vi "Mini-Circuits-RF-Switch.vi"(6 "RFSW State":T1=enum."1", 7 "RFSW Letter":T2, 11 "Switch 1 SN":string(combo)) -> (0 "Error Out":errorcluster, 3 "SWA":bool, 4 "Model_Name SW1":string)   [LabVIEW 2020]
uses:
  Subs/RFSW Letter.ctl
  Subs/RFSW State.ctl
  Subs/Mini-Circuits-RF-Switch.ctl
  <vilib>/Utility/file.llb/Read Delimited Spreadsheet (string).vi
  <vilib>/Utility/file.llb/Write Delimited Spreadsheet (string).vi
panel:
  out "ExeName":string
  out "Test Config Path Out":path
  in  "Set_Switch":bool
  out "current test path":string[](array[string])
  out "test-paths":string[](array[string])=["CMN4-RX1", "CMN4-RX2", "CMN4-NF1", "CMN4-NF2", "UVL-TX1", "UVL-TX2", "WBHD-RX1", "WBHD-RX2", "WBHD-RX3", "WBHD-NF1", "WBHD-NF2", "WBHD-NF3", "WBHD-TX1", "WBHD-TX2", "WBHD-TX3", "NB-RX1", "NB-RX2", "NB-NF1", "NB-NF2"]
  out "State":string="Exit"
  out "INI Path":path=path "C:/Users/J54147.NORTHGRUM/OneDrive - NGC/Documents/LabVIEW Data/Config Files/mcl_RF_Switch_Main_GUI_Config.ini"
  in  "Tab Control":enum32{"Main", "Configuration"}(tab)
  in  "Stop Button":bool
  in  "Load Config":bool
  in  "Save Config":bool
  in  "Get_State":bool
  in  "Set Path":bool
  in  "Test Path":T3
  in  "Switch 2 SN":string(combo)
  out "Model_Name SW2":string
  out "SW B":bool
  in  "SW 2A":u8(knob)=1 min=1 max=7 step=1 scale=1.0..6.0
  in  "SW 1B":u8(knob)=1 min=1 max=7 step=1 scale=1.0..6.0
  in  "SW 1A":u8(knob)=1 min=1 max=7 step=1 scale=1.0..6.0
  in  "Paths Config":string[][](table)
  in  "Test Config Path":path
  # "AMCTR RF SWITCH UTILITY"
  # "v.1.0"
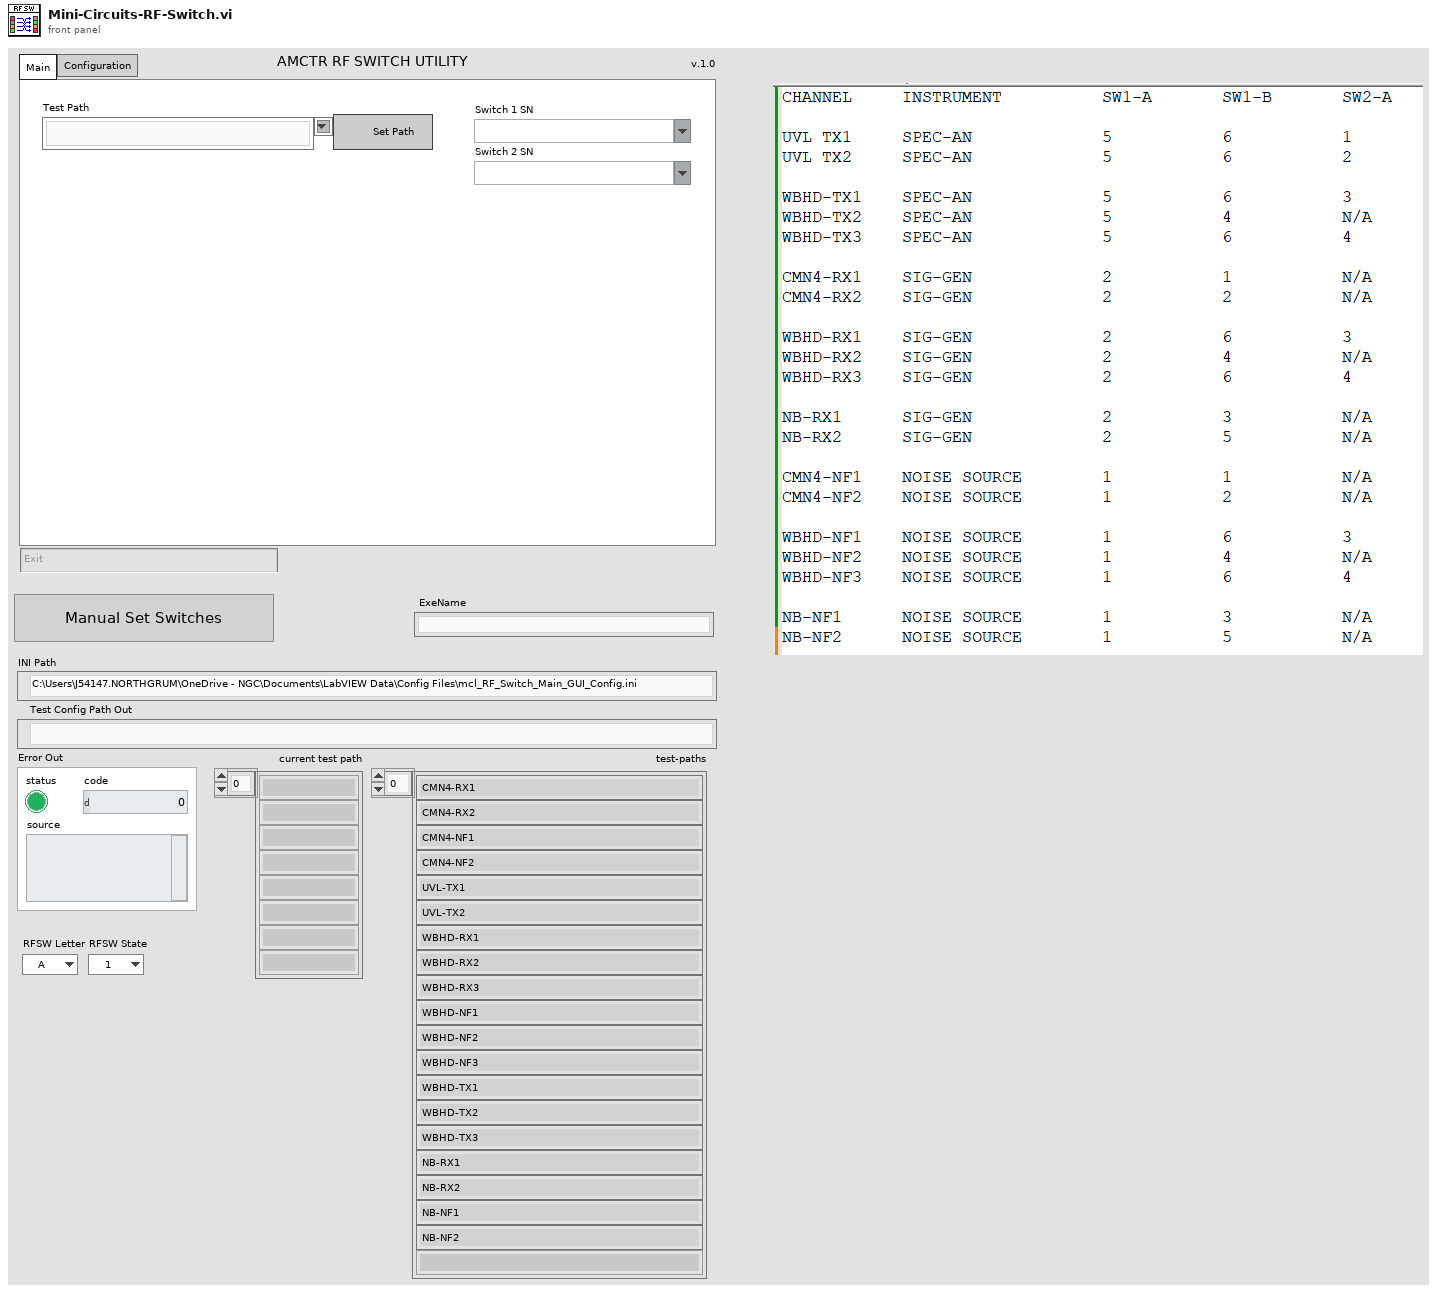
[diagram p1: front panel]
types:
  T1 = typedef "RFSW State.ctl" = enum16{"0", "1", "2", "3", "4", "5", "6"}
  T2 = typedef "RFSW Letter.ctl" = enum16{"A", "B"}
  T3 = typedef "Mini-Circuits-RF-Switch.ctl" = string
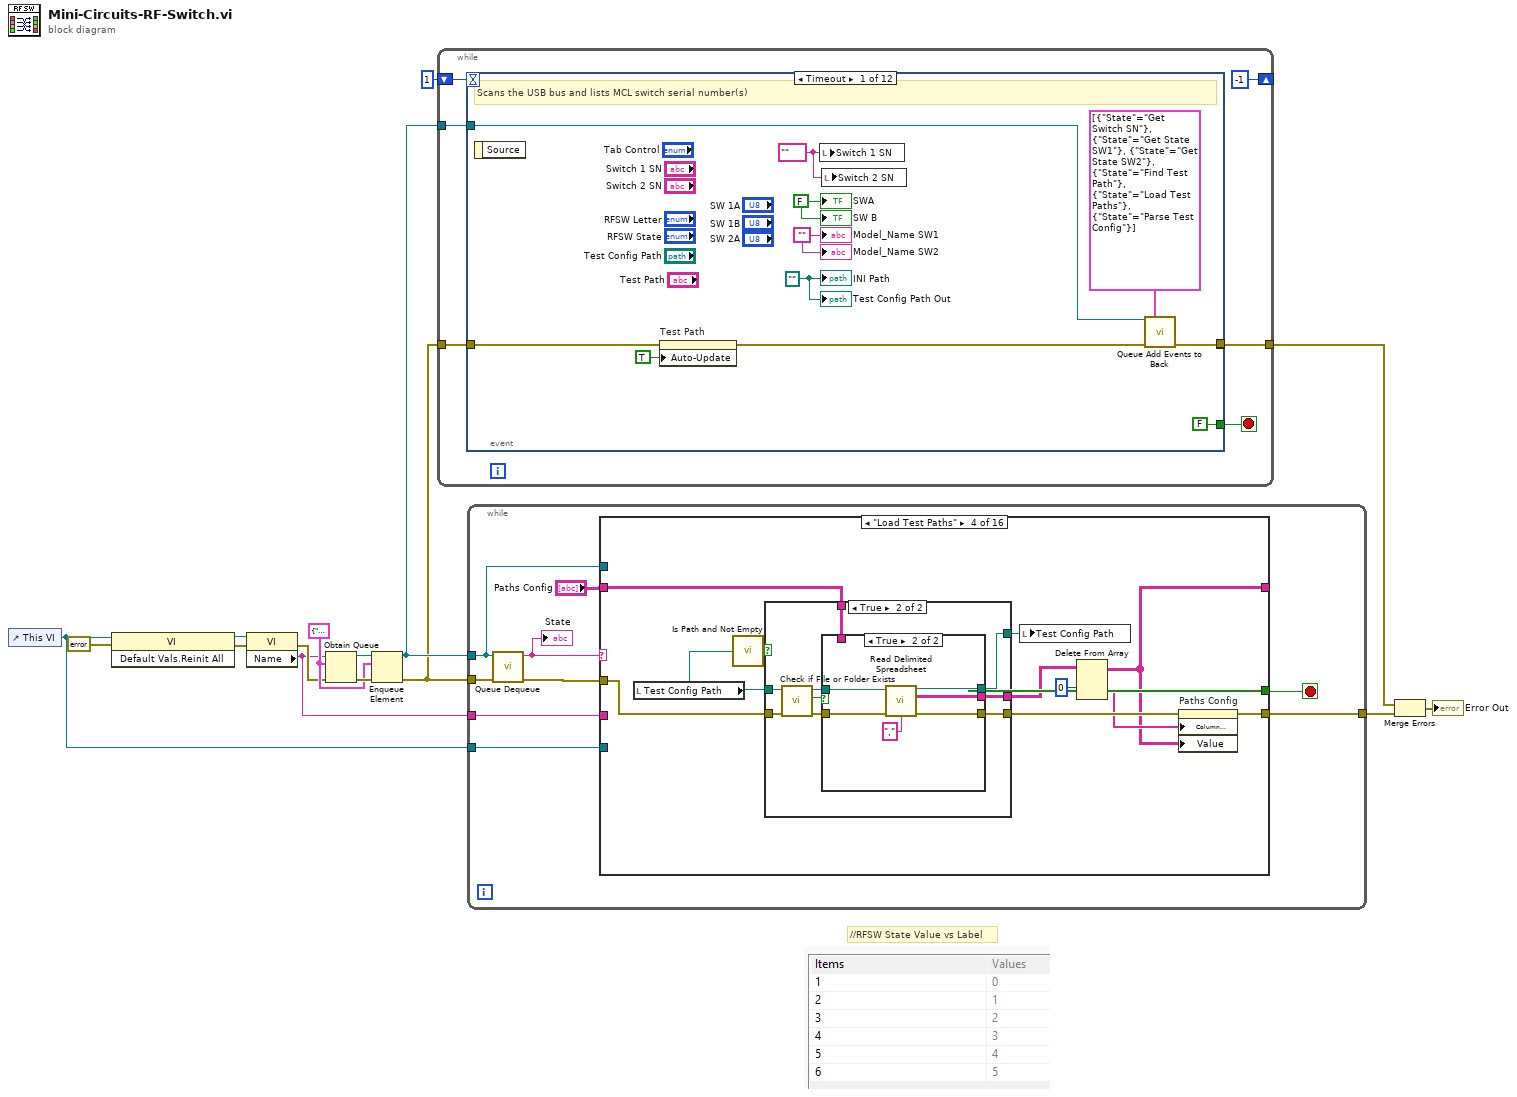
[diagram p0: block diagram]
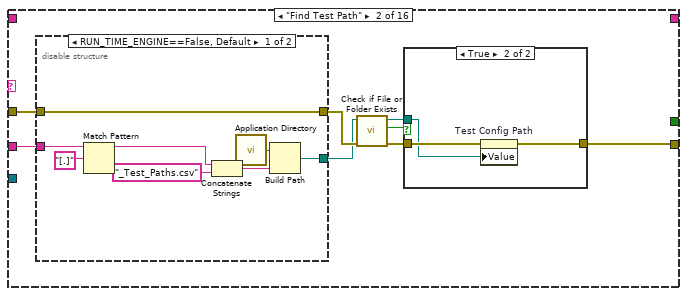
[diagram p3: hidden frame]
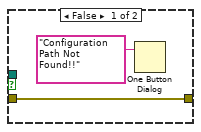
[diagram p4: hidden frame]
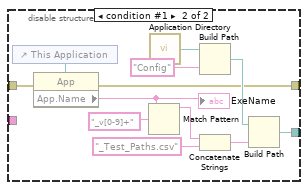
[diagram p5: hidden frame]
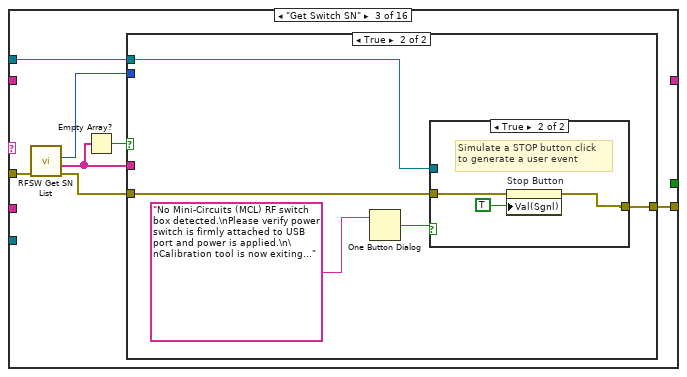
[diagram p6: hidden frame]
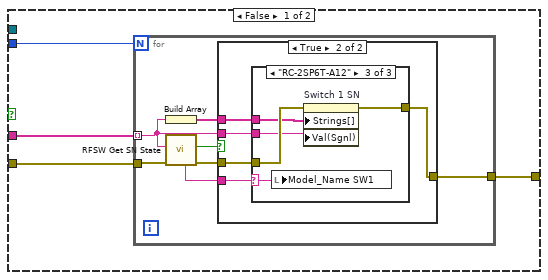
[diagram p7: hidden frame]
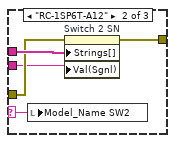
[diagram p10: hidden frame]
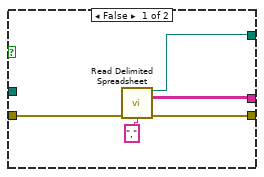
[diagram p12: hidden frame]
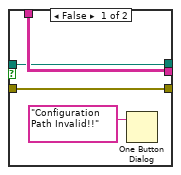
[diagram p13: hidden frame]
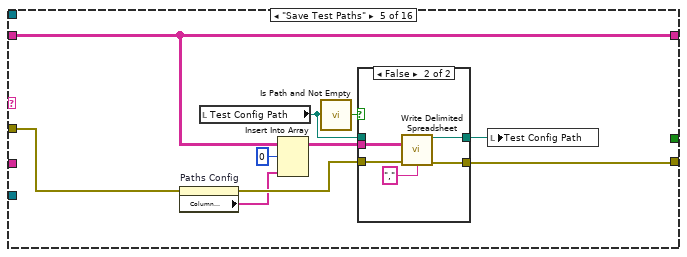
[diagram p14: hidden frame]
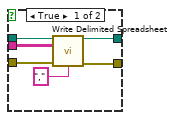
[diagram p15: hidden frame]
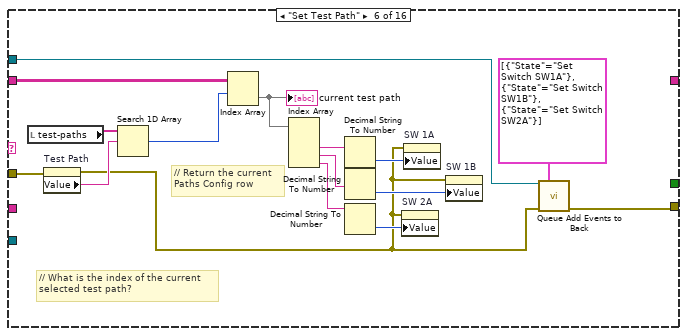
[diagram p16: hidden frame]
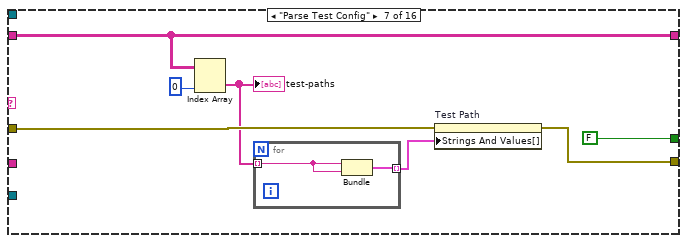
[diagram p17: hidden frame]
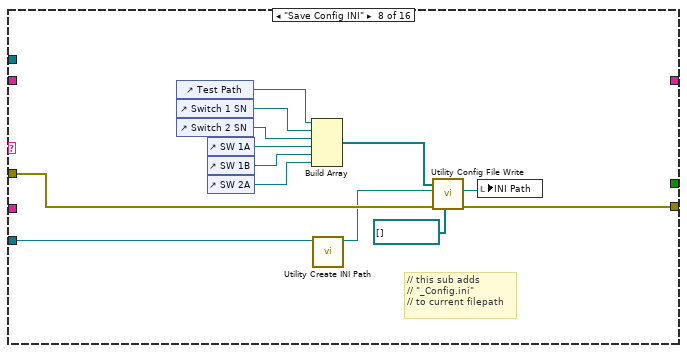
[diagram p18: hidden frame]
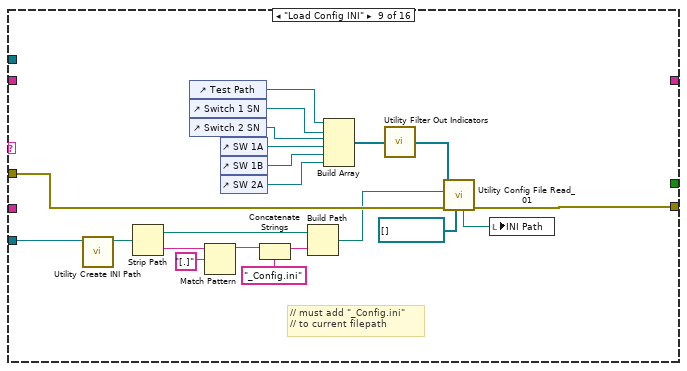
[diagram p19: hidden frame]
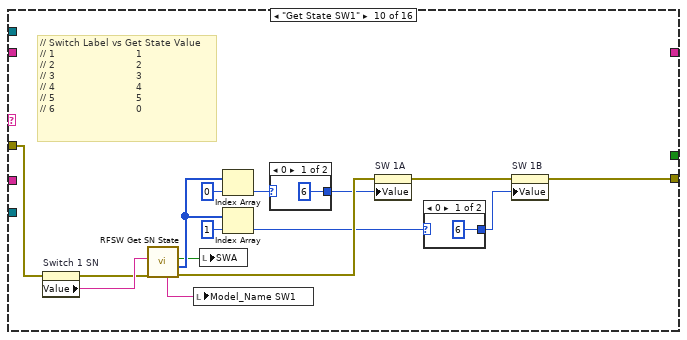
[diagram p20: hidden frame]
diagram:
  w11 = cluster{"State":string, "Data":variant} {"State"="", "Data"=variant} ("Cluster")
  # "//RFSW State Value vs Label"
  n1 = control-ref of="This VI"() -> (w4:refnum<vi>)
  n2 = invoke class="VI" method="Default Vals.Reinit All"(reference=w4, error in=errorcluster {"status"=FALSE, "code"=0, "source"=""} ("Error In")) -> (reference out=w8:refnum<vi>, error out=w7:errorcluster)  [unwired: 1 in, 1 out]
  n3 = property class="VI"(reference=w8, error in=w7) -> (error out=w10:errorcluster, "Name"=w1:string)  [unwired: 1 out]
  n4 = Obtain Queue(name (unnamed)=w1, element data type=w11, error in (no error)=w10) -> (queue out=w12:refnum<queue>, error out=w13:errorcluster)  [unwired: 2 in, 1 out]
  n5 = Enqueue Element(queue=w12, element=w11, error in (no error)=w13) -> (queue out=w9:refnum<queue>, error out=w2:errorcluster)  [unwired: 1 in, 1 out]
  n6 = while {
    tunnel: w2 -> [w21]
    tunnel: [w20] -> w15
    shift-right: [-1] -> _
    shift-left: 1 -> [w18]
    tunnel: w9 -> [w16]
    stop <- w19 stop-if-true
    n7 = event shown="[0] Timeout" {
      selector: _ -> [_ _ _ _ _ _ _ _ _ _ _ _]
      dyn-events: _ -> [_ _ _ _ _ _ _ _ _ _ _ _]
      timeout: w18 -> [_ _ _ _ _ _ _ _ _ _ _ _]
      tunnel: w21 -> [w24 w35 w44 w52 w58 w69 w73 w77 w81 w85 w91 w103]
      tunnel: [_ w34 w43 w51 w57 w68 w71 w75 w79 w84 w90 w102] -> w20
      tunnel: [FALSE _ _ FALSE FALSE FALSE _ _ _ TRUE TRUE TRUE] -> w19
      tunnel: w16 -> [w29 w36 w45 w53 w59 w66 w72 w76 w80 w86 w92 w104]
      tunnel: [w28 _ _ _ _ _ _ _ _ _ _ _] -> _
      event Timeout {
        w25 = "" ("Switch 1 SN")
        w26 = path ""
        w30 = ""
        w31 = FALSE ("Connected?")
        # "Scans the USB bus and lists MCL switch serial number(s)"
        n8 = event-data() -> ()  [unwired: 1 in, 1 out]
        n9 = property on="Test Path" class="CmbBox (strict)"(error in=w24, "Auto-Update"=TRUE ("Auto-Update From Typedef")) -> (error out=w23:errorcluster)  [unwired: 1 in, 1 out]
        n10 = local write "Switch 1 SN"(w25) -> ()
        n11 = local write "Switch 2 SN"(w25) -> ()
        n12 = call "Queue Add Events to Back.vi"("Queue In"=w29, "State Array"=cluster{"State":string}[] [{"State"="Get Switch SN"}, {"State"="Get State SW1"}, {"State"="Get State SW2"}, {"State"="Find Test Path"}, {"State"="Load Test Paths"}, {"State"="Parse Test Config"}], "Error In"=w23) -> ("Error Out"=w28:errorcluster)  [unwired: 11 in, 1 out]
        "Model_Name SW1" <- w30
        "SWA" <- w31
        "INI Path" <- w26
        "SW B" <- w31
        "Model_Name SW2" <- w30
        "Test Config Path Out" <- w26
      }
      event "Save Config": Value Change {
        n13 = event-data() -> ("NewVal"=w33:bool)  [unwired: 1 in]
        n14 = case shown="True" w33 {
          tunnel: w36 -> [_ w40]
          tunnel: w35 -> [w37 w39]
          tunnel: [w37 w38] -> w34
          frame False {
          }
          frame True {
            n15 = call "Queue Add Events to Back.vi"("Queue In"=w40, "State Array"=cluster{"State":string}[] [{"State"="Save Config INI"}, {"State"="Save Test Paths"}], "Error In"=w39) -> ("Error Out"=w38:errorcluster)  [unwired: 11 in, 1 out]
          }
        }
      }
      event "Load Config": Value Change {
        n16 = event-data() -> ("NewVal"=w42:bool)  [unwired: 1 in]
        n17 = case shown="True" w42 {
          tunnel: w45 -> [_ w49]
          tunnel: w44 -> [w46 w48]
          tunnel: [w46 w47] -> w43
          frame False {
          }
          frame True {
            n18 = call "Queue Add Events to Back.vi"("Queue In"=w49, "State Array"=cluster{"State":string}[] [{"State"="Load Config INI"}], "Error In"=w48) -> ("Error Out"=w47:errorcluster)  [unwired: 11 in, 1 out]
          }
        }
      }
      event "Set_Switch": Value Change {
        n19 = event-data() -> ()  [unwired: 1 in, 1 out]
        n20 = call "Queue Add Events to Back.vi"("Queue In"=w53, "State Array"=cluster{"State":string}[] [{"State"="Set Switch SW1A"}, {"State"="Set Switch SW1B"}, {"State"="Set Switch SW2A"}], "Error In"=w52) -> ("Error Out"=w51:errorcluster)  [unwired: 11 in, 1 out]
      }
      event "Set Path": Value Change {
        n21 = event-data() -> ("NewVal"=w56:bool)  [unwired: 1 in]
        n22 = case shown="True" w56 {
          tunnel: w59 -> [_ w64]
          tunnel: w58 -> [w61 w63]
          tunnel: [w61 w62] -> w57
          frame False {
          }
          frame True {
            n23 = call "Queue Add Events to Back.vi"("Queue In"=w64, "State Array"=cluster{"State":string}[] [{"State"="Set Test Path"}], "Error In"=w63) -> ("Error Out"=w62:errorcluster)  [unwired: 11 in, 1 out]
          }
        }
      }
      event "Get_State": Value Change {
        n24 = event-data() -> ()  [unwired: 1 in, 1 out]
        n25 = call "Queue Add Events to Back.vi"("Queue In"=w66, "State Array"=cluster{"State":string}[] [{"State"="Get State SW1"}, {"State"="Get State SW2"}], "Error In"=w69) -> ("Error Out"=w68:errorcluster)  [unwired: 11 in, 1 out]
      }
      event "SW 1A": Value Change {
        n26 = event-data() -> ()  [unwired: 1 in, 1 out]
        n27 = call "Queue Add Events to Back.vi"("Queue In"=w72, "State Array"=cluster{"State":string}[] [{"State"="Set Switch SW1A"}], "Error In"=w73) -> ("Error Out"=w71:errorcluster)  [unwired: 11 in, 1 out]
      }
      event "SW 1B": Value Change {
        n28 = event-data() -> ()  [unwired: 1 in, 1 out]
        n29 = call "Queue Add Events to Back.vi"("Queue In"=w76, "State Array"=cluster{"State":string}[] [{"State"="Set Switch SW1B"}], "Error In"=w77) -> ("Error Out"=w75:errorcluster)  [unwired: 11 in, 1 out]
      }
      event "SW 2A": Value Change {
        n30 = event-data() -> ()  [unwired: 1 in, 1 out]
        n31 = call "Queue Add Events to Back.vi"("Queue In"=w80, "State Array"=cluster{"State":string}[] [{"State"="Set Switch SW2A"}], "Error In"=w81) -> ("Error Out"=w79:errorcluster)  [unwired: 11 in, 1 out]
      }
      event Panel Close? {
        n32 = event-data() -> ()  [unwired: 1 in, 1 out]
        n33 = call "Queue Add Events to Back.vi"("Queue In"=w86, "State Array"=cluster{"State":string}[] [{"State"="Save Config INI"}, {"State"="Save Test Paths"}, {"State"="Exit"}], "Error In"=w85) -> ("Error Out"=w84:errorcluster)  [unwired: 11 in, 1 out]
        n34 = event-data("Discard?"=TRUE) -> ()  [unwired: 1 in, 1 out]
      }
      event "Stop Button": Value Change {
        n35 = event-data() -> ("NewVal"=w89:bool)  [unwired: 1 in]
        n36 = case shown="True" w89 {
          tunnel: w92 -> [_ w100]
          tunnel: w91 -> [w94 w99]
          tunnel: [w94 w96] -> w90
          frame False {
          }
          frame True {
            n37 = call "Queue Add Events to Back.vi"("Queue In"=w100, "State Array"=cluster{"State":string}[] [{"State"="Save Config INI"}, {"State"="Save Test Paths"}, {"State"="Exit"}], "Error In"=w99) -> ("Error Out"=w97:errorcluster)  [unwired: 11 in, 1 out]
            n38 = property on="Stop Button" class="Bool (strict)"(error in=w97, "Value"=FALSE ("Stop Button")) -> (error out=w96:errorcluster)  [unwired: 1 in, 1 out]
          }
        }
      }
      event Application Instance Close {
        n39 = event-data() -> ()  [unwired: 1 in, 1 out]
        n40 = call "Queue Add Events to Back.vi"("Queue In"=w104, "State Array"=cluster{"State":string}[] [{"State"="Save Config INI"}, {"State"="Save Test Paths"}, {"State"="Exit"}], "Error In"=w103) -> ("Error Out"=w102:errorcluster)  [unwired: 11 in, 1 out]
      }
    }
  }
  n41 = while {
    tunnel: w2 -> [w114]
    tunnel: w9 -> [w110]
    tunnel: w4 -> [w109]
    tunnel: [w107] -> w5
    tunnel: w1 -> [w106]
    stop <- w112 stop-if-true
    n42 = call "Queue Dequeue.vi"("Error In"=w114, "Queue In"=w110) -> ("Error Out"=w111:errorcluster, "State"=w113:string)  [unwired: 7 in, 1 out]
    "State" <- w113
    n43 = case shown="\"Load Test Paths\"" w113 {
      tunnel: "Paths Config" -> [_ _ _ w197 w237 w261 w266 _ _ _ _ _ _ _ _ _]
      tunnel: [_ _ _ _ _ _ FALSE _ _ _ _ _ _ _ _ w384] -> w112
      tunnel: w111 -> [w115 w123 w155 w198 w235 w264 w269 w286 w307 w313 w330 w344 w352 w365 w373 w382]
      tunnel: w110 -> [_ _ w149 _ _ w250 _ _ _ _ _ _ _ _ _ w385]
      tunnel: w109 -> [_ _ _ _ _ _ _ w285 w306 _ _ _ _ _ _ _]
      tunnel: [_ _ _ w193 w237 _ w266 _ _ _ _ _ _ _ _ _] -> _
      tunnel: [w115 w122 w152 w200 w236 w249 w265 w284 w305 w308 w327 w341 w351 w362 w372 w383] -> w107
      tunnel: w106 -> [_ w121 _ _ _ _ _ _ _ _ _ _ _ _ _ _]
      frame "Timeout", Default {
      }
      frame "Find Test Path" {
        n44 = disable-structure shown="RUN_TIME_ENGINE==False, Default" {
          disable-tunnel: w121 -> [w131 _]
          disable-tunnel: [w134 w146] -> w118
          disable-tunnel: w123 -> [w129 w139]
          disable-tunnel: [w129 w137] -> w120
          frame condition #0 (active) {
            n45 = Match Pattern(string=w131, regular expression="[.]" ("search string")) -> (before substring=w130:string)  [unwired: 1 in, 3 out]
            n46 = Concatenate Strings(w130, "_Test_Paths.csv" ("string")) -> (w136:string)
            n47 = call <vilib>:"Application Directory.vi"() -> ("Application Directory"=w133:path)
            n48 = Build Path(base path=w133, name or relative path=w136) -> (appended path=w134:path)
          }
          frame condition #1 {
            n49 = control-ref of="This Application"() -> (w138:refnum<vi>)
            n50 = property class="App"(reference=w138, error in=w139) -> (error out=w137:errorcluster, "App.Name"=w140:string)  [unwired: 1 out]
            "ExeName" <- w140
            n51 = Match Pattern(string=w140, regular expression="_v[0-9]+" ("search string")) -> (before substring=w141:string)  [unwired: 1 in, 3 out]
            n52 = call <vilib>:"Application Directory.vi"() -> ("Application Directory"=w145:path)
            n53 = Build Path(base path=w145, name or relative path="Config") -> (appended path=w143:path)
            n54 = Concatenate Strings(w141, "_Test_Paths.csv" ("string")) -> (w148:string)
            n55 = Build Path(base path=w143, name or relative path=w148) -> (appended path=w146:path)
          }
        }
        n56 = call <vilib>:"Check if File or Folder Exists.vi"("error in (no error)"=w120, "path"=w118) -> ("error out"=w119:errorcluster, "file or folder exists?"=w117:bool, "dup path"=w116:path)  [unwired: 7 in]
        n57 = case shown="True" w117 {
          tunnel: [w125 w128] -> w122
          tunnel: w119 -> [w125 w127]
          tunnel: w116 -> [_ w126]
          frame False {
            n58 = One Button Dialog(message="Configuration Path Not Found!!") -> ()  [unwired: 1 in, 1 out]
          }
          frame True {
            n59 = property on="Test Config Path" class="Path"(error in=w127, "Value"=w126) -> (error out=w128:errorcluster)  [unwired: 1 in, 1 out]
          }
        }
      }
      frame "Get Switch SN" {
        n60 = call "RFSW Get SN List.vi"("Error_In"=w155) -> ("Error_Out"=w154:errorcluster, "SN_Array"=w151:string[], "Num_Switches"=w153:i32)  [unwired: 7 in, 1 out]
        n61 = Empty Array?(array=w151) -> (empty?=w150:bool)
        n62 = case shown="True" w150 {
          tunnel: w154 -> [w159 w186]
          tunnel: w153 -> [w158 _]
          tunnel: [w157 w188] -> w152
          tunnel: w151 -> [w156 _]
          tunnel: w149 -> [_ w187]
          frame False {
            n63 = for {
              N: w158 -> [_]
              tunnel: w156 -> [w160] mode=indexing
              tunnel: w159 -> [w165]
              tunnel: [w163] -> w157
              n64 = Build Array(w160) -> (w166:string[])
              n65 = call "RFSW Get SN State.vi"("error in (no error)"=w165, "SN"=w160) -> ("error out"=w164:errorcluster, "Connected?"=w161:bool, "Model Name"=w162:string)  [unwired: 5 in, 2 out]
              n66 = case shown="True" w161 {
                tunnel: w166 -> [_ w172]
                tunnel: w164 -> [w167 w171]
                tunnel: [w167 w170] -> w163
                tunnel: w162 -> [_ w169]
                tunnel: w160 -> [_ w168]
                frame False {
                }
                frame True {
                  n67 = case shown="\"RC-2SP6T-A12\"" w169 {
                    selector: w169 -> [_ w178 w183]
                    tunnel: w172 -> [_ w177 w181]
                    tunnel: w171 -> [w173 w176 w182]
                    tunnel: [w173 w175 w180] -> w170
                    tunnel: w168 -> [_ w174 w179]
                    frame Default {
                    }
                    frame "RC-1SP6T-A12" {
                      n68 = local write "Model_Name SW2"(w178) -> ()
                      n69 = property on="Switch 2 SN" class="CmbBox"(error in=w176, "Strings[]"=w177, "Val(Sgnl)"=w174) -> (error out=w175:errorcluster)  [unwired: 1 in, 1 out]
                    }
                    frame "RC-2SP6T-A12" {
                      n70 = local write "Model_Name SW1"(w183) -> ()
                      n71 = property on="Switch 1 SN" class="CmbBox"(error in=w182, "Strings[]"=w181, "Val(Sgnl)"=w179) -> (error out=w180:errorcluster)  [unwired: 1 in, 1 out]
                    }
                  }
                }
              }
            }
          }
          frame True {
            n72 = One Button Dialog(message="No Mini-Circuits (MCL) RF switch box detected.\nPlease verify power switch is firmly attached to USB port and power is applied.\n\nCalibration tool is now exiting...") -> (true=w185:bool)  [unwired: 1 in]
            n73 = case shown="True" w185 {
              tunnel: [w189 w191] -> w188
              tunnel: w187 -> [_ _]
              tunnel: w186 -> [w189 w192]
              frame False {
              }
              frame True {
                # "Simulate a STOP button click\nto generate a user event"
                n74 = property on="Stop Button" class="Bool (strict)"(error in=w192, "Val(Sgnl)"=TRUE ("Value (Signaling)")) -> (error out=w191:errorcluster)  [unwired: 1 in, 1 out]
              }
            }
          }
        }
      }
      frame "Load Test Paths" {
        n75 = local read "Test Config Path"() -> (w195:path)
        n76 = call <vilib>:"Is Path and Not Empty.vi"("path"=w195) -> ("Is Path and Not Empty?"=w196:bool)  [unwired: 4 in]
        n77 = case shown="True" w196 {
          tunnel: [w205 w217] -> w203
          tunnel: [w206 w216] -> w201
          tunnel: w198 -> [w207 w215]
          tunnel: w197 -> [_ w212]
          tunnel: w195 -> [_ w211]
          tunnel: [w204 w209] -> w194
          frame False {
            n78 = call-poly <vilib>:"Read Delimited Spreadsheet.vi"("error in (no error)"=w207, "delimiter (\\t)"="," ("delimiter (\\t)")) -> ("new file path (Not A Path if cancelled)"=w204:path, "all rows"=w205:string[][], "error out"=w206:errorcluster)  [unwired: 8 in, 3 out]
          }
          frame True {
            n79 = call <vilib>:"Check if File or Folder Exists.vi"("error in (no error)"=w215, "path"=w211) -> ("error out"=w214:errorcluster, "file or folder exists?"=w213:bool, "dup path"=w210:path)  [unwired: 7 in]
            n80 = case shown="True" w213 {
              tunnel: [w220 w226] -> w217
              tunnel: [w221 w225] -> w216
              tunnel: w214 -> [w221 w224]
              tunnel: w212 -> [w220 _]
              tunnel: w210 -> [w218 w223]
              tunnel: [w218 w222] -> w209
              frame False {
                n81 = One Button Dialog(message="Configuration Path Invalid!!") -> ()  [unwired: 1 in, 1 out]
              }
              frame True {
                n82 = call-poly <vilib>:"Read Delimited Spreadsheet.vi"("file path (dialog if empty)"=w223, "error in (no error)"=w224, "delimiter (\\t)"="," ("delimiter (\\t)")) -> ("new file path (Not A Path if cancelled)"=w222:path, "all rows"=w226:string[][], "error out"=w225:errorcluster)  [unwired: 7 in, 3 out]
              }
            }
          }
        }
        n83 = local write "Test Config Path"(w194) -> ()
        n84 = Delete From Array(array=w203, index (row)=0) -> (deleted portion=w199:string[], array with subset deleted=w193:string[][])  [unwired: 2 in]
        n85 = property on="Paths Config" class="Tbl (strict)"(error in=w201, "Column Headers[]"=w199, "Value"=w193) -> (error out=w200:errorcluster)  [unwired: 1 in, 1 out]
      }
      frame "Save Test Paths" {
        n86 = property on="Paths Config" class="Tbl (strict)"(error in=w235) -> (error out=w233:errorcluster, "Column Headers[]"=w232:string[])  [unwired: 1 in, 1 out]
        n87 = local read "Test Config Path"() -> (w234:path)
        n88 = Insert Into Array(array=w237, index (row)=0, new element=w232) -> (w230:string[][])  [unwired: 1 in]
        n89 = call <vilib>:"Is Path and Not Empty.vi"("path"=w234) -> ("Is Path and Not Empty?"=w229:bool)  [unwired: 4 in]
        n90 = case shown="False" w229 {
          tunnel: [w243 w248] -> w236
          tunnel: w234 -> [w242 _]
          tunnel: w233 -> [w240 w246]
          tunnel: w230 -> [w239 w245]
          tunnel: [w238 w244] -> w228
          frame True {
            n91 = call-poly <vilib>:"Write Delimited Spreadsheet.vi"("file path (dialog if empty)"=w242, "2D data"=w239, "error in (no error)"=w240, "delimiter (\\t)"="," ("delimiter (\\t)")) -> ("new file path (Not A Path if cancelled)"=w238:path, "error out"=w243:errorcluster)  [unwired: 10 in]
          }
          frame False {
            n92 = call-poly <vilib>:"Write Delimited Spreadsheet.vi"("2D data"=w245, "error in (no error)"=w246, "delimiter (\\t)"="," ("delimiter (\\t)")) -> ("new file path (Not A Path if cancelled)"=w244:path, "error out"=w248:errorcluster)  [unwired: 11 in]
          }
        }
        n93 = local write "Test Config Path"(w228) -> ()
      }
      frame "Set Test Path" {
        # "// Return the current\nPaths Config row"
        # "// What is the index of the current\nselected test path?"
        n94 = local read "test-paths"() -> (w263:string[])
        n95 = property on="Test Path" class="CmbBox (strict)"(error in=w264) -> (error out=w251:errorcluster, "Value"=w262:T3)  [unwired: 1 in, 1 out]
        n96 = Search 1D Array(1D array=w263, element=w262) -> (index of element=w260:i32)  [unwired: 1 in]
        n97 = Index Array(array=w261, index (row)=w260) -> (element=w259:string[])  [unwired: 1 in]
        "current test path" <- w259
        n98 = Index Array(array=w259) -> (element #2=w258:string, element #3=w256:string, element #4=w254:string)  [unwired: 4 in, 1 out]
        n99 = Decimal String To Number(string=w258) -> (number=w257:i32)  [unwired: 2 in, 1 out]
        n100 = Decimal String To Number(string=w256) -> (number=w255:i32)  [unwired: 2 in, 1 out]
        n101 = Decimal String To Number(string=w254) -> (number=w253:i32)  [unwired: 2 in, 1 out]
        n102 = property on="SW 2A" class="Knob (strict)"(error in=w251, "Value"=w253) -> ()  [unwired: 1 in, 2 out]
        n103 = property on="SW 1A" class="Knob (strict)"(error in=w251, "Value"=w257) -> ()  [unwired: 1 in, 2 out]
        n104 = property on="SW 1B" class="Knob (strict)"(error in=w251, "Value"=w255) -> ()  [unwired: 1 in, 2 out]
        n105 = call "Queue Add Events to Back.vi"("Queue In"=w250, "State Array"=cluster{"State":string}[] [{"State"="Set Switch SW1A"}, {"State"="Set Switch SW1B"}, {"State"="Set Switch SW2A"}], "Error In"=w251) -> ("Error Out"=w249:errorcluster)  [unwired: 11 in, 1 out]
      }
      frame "Parse Test Config" {
        n106 = Index Array(array=w266, index (col)=0 ("index")) -> (element=w268:string[])  [unwired: 1 in]
        "test-paths" <- w268
        n107 = for {
          tunnel: w268 -> [w273] mode=indexing
          tunnel: [w272] -> w267 mode=indexing
          n108 = Bundle(w273, w273) -> (w272:cluster{string, string})  [unwired: 1 in]
        }
        n109 = property on="Test Path" class="CmbBox (strict)"(error in=w269, "Strings And Values[]"=w267) -> (error out=w265:errorcluster)  [unwired: 1 in, 1 out]
      }
      frame "Save Config INI" {
        # "// this sub adds\n// \"_Config.ini\"\n// to current filepath"
        n110 = control-ref of="Test Path"() -> (w279:refnum<vi>)
        n111 = control-ref of="Switch 1 SN"() -> (w283:refnum<vi>)
        n112 = control-ref of="Switch 2 SN"() -> (w280:refnum<vi>)
        n113 = control-ref of="SW 1A"() -> (w278:refnum<vi>)
        n114 = control-ref of="SW 1B"() -> (w277:refnum<vi>)
        n115 = control-ref of="SW 2A"() -> (w276:refnum<vi>)
        n116 = Build Array(w279, w283, w280, w278, w277, w276) -> (w282:refnum<vi>[])
        n117 = call "Utility Create INI Path.vi"("VI Ref In"=w285) -> ("INI Path"=w274:path)  [unwired: 10 in]
        n118 = call "Utility Config File Write.vi"("Controls Excluded"=refnum<vi>[] [], "Error In"=w286, "Path"=w274, "Controls In"=w282) -> ("Error Out"=w284:errorcluster, "Path_Out"=w275:path)  [unwired: 6 in]
        n119 = local write "INI Path"(w275) -> ()
      }
      frame "Load Config INI" {
        # "// must add \"_Config.ini\"\n// to current filepath"
        n120 = call "Utility Create INI Path.vi"("VI Ref In"=w306) -> ("INI Path"=w294:path)  [unwired: 10 in]
        n121 = Strip Path(path=w294) -> (stripped path=w288:path, name=w293:string)
        n122 = control-ref of="Test Path"() -> (w296:refnum<vi>)
        n123 = control-ref of="Switch 1 SN"() -> (w297:refnum<vi>)
        n124 = control-ref of="Switch 2 SN"() -> (w298:refnum<vi>)
        n125 = Match Pattern(string=w293, regular expression="[.]" ("search string")) -> (before substring=w291:string)  [unwired: 1 in, 3 out]
        n126 = control-ref of="SW 1A"() -> (w304:refnum<vi>)
        n127 = control-ref of="SW 1B"() -> (w300:refnum<vi>)
        n128 = control-ref of="SW 2A"() -> (w299:refnum<vi>)
        n129 = Concatenate Strings(w291, "_Config.ini") -> (w289:string)
        n130 = Build Path(base path=w288, name or relative path=w289) -> (appended path=w287:path)
        n131 = Build Array(w296, w297, w298, w304, w300, w299) -> (w301:refnum<vi>[])
        n132 = call "Utility Filter Out Indicators.vi"("Controls In"=w301) -> ("Controls Out"=w303:refnum<vi>[])
        n133 = call "Utility Config File Read_01.vi"("Controls Excluded"=refnum<vi>[] [], "Error In"=w307, "Path"=w287, "Controls In"=w303) -> ("Error Out"=w305:errorcluster, "Path_Out"=w295:path)  [unwired: 3 in, 3 out]
        n134 = local write "INI Path"(w295) -> ()
      }
      frame "Get State SW1" {
        # "// Switch Label vs Get State Value\n// 1                           1\n// 2                           2\n// 3                           3\n// 4                           4\n// 5                           5\n// 6                           0"
        n135 = property on="Switch 1 SN" class="CmbBox"(error in=w313) -> (error out=w314:errorcluster, "Value"=w315:string)  [unwired: 1 in, 1 out]
        n136 = call "RFSW Get SN State.vi"("error in (no error)"=w314, "SN"=w315) -> ("error out"=w321:errorcluster, "PortAB_Array"=w318:i32[], "Connected?"=w317:bool, "Model Name"=w316:string)  [unwired: 5 in, 1 out]
        n137 = local write "Model_Name SW1"(w316) -> ()
        n138 = local write "SWA"(w317) -> ()
        n139 = Index Array(array=w318, index=0) -> (element=w310:i32)
        n140 = Index Array(array=w318, index=1) -> (element=w312:i32)
        n141 = case shown="0" w310 {
          selector: w310 -> [_ w324]
          tunnel: [6 w324] -> w309
          frame 0 {
          }
          frame 1..5, Default {
          }
        }
        n142 = property on="SW 1A" class="Knob (strict)"(error in=w321, "Value"=w309) -> (error out=w322:errorcluster)  [unwired: 1 in, 1 out]
        n143 = case shown="0" w312 {
          selector: w312 -> [_ w326]
          tunnel: [6 w326] -> w311
          frame 0 {
          }
          frame 1..5, Default {
          }
        }
        n144 = property on="SW 1B" class="Knob (strict)"(error in=w322, "Value"=w311) -> (error out=w308:errorcluster)  [unwired: 1 in, 1 out]
      }
      frame "Get State SW2" {
        # "// Switch Label vs Get State Value\n// 1                           1\n// 2                           2\n// 3                           3\n// 4                           4\n// 5                           5\n// 6                           0"
        n145 = property on="Switch 2 SN" class="CmbBox"(error in=w330) -> (error out=w336:errorcluster, "Value"=w337:string)  [unwired: 1 in, 1 out]
        n146 = call "RFSW Get SN State.vi"("error in (no error)"=w336, "SN"=w337) -> ("error out"=w333:errorcluster, "PortAB_Array"=w332:i32[], "Connected?"=w334:bool, "Model Name"=w335:string)  [unwired: 5 in, 1 out]
        n147 = local write "SW B"(w334) -> ()
        n148 = local write "Model_Name SW2"(w335) -> ()
        n149 = Index Array(array=w332, index=0) -> (element=w329:i32)
        n150 = case shown="1..5, Default" w329 {
          selector: w329 -> [_ w339]
          tunnel: [6 w339] -> w328
          frame 0 {
          }
          frame 1..5, Default {
          }
        }
        n151 = property on="SW 2A" class="Knob (strict)"(error in=w333, "Value"=w328) -> (error out=w327:errorcluster)  [unwired: 1 in, 1 out]
      }
      frame "Set Switch SW1A" {
        n152 = property on="Switch 1 SN" class="CmbBox"(error in=w344) -> (error out=w343:errorcluster, "Value"=w346:string)  [unwired: 1 in, 1 out]
        n153 = property on="SW 1A" class="Knob (strict)"(error in=w343) -> (error out=w342:errorcluster, "Value"=w340:u8)  [unwired: 1 in, 1 out]
        n154 = call "RFSW Set.vi"("RFSW State"=w340, "RFSW Letter"=RFSW_Letter."A", "error in (no error)"=w342, "SN"=w346) -> ("error out"=w341:errorcluster)  [unwired: 4 in, 3 out]
      }
      frame "Set Switch SW1B" {
        n155 = local read "Model_Name SW1"() -> (w350:string)
        n156 = Match True/False String(2:"" ("false string"), 3:"RC-2SP6T" ("true string"), 4:w350) -> (0:w347:bool)  [unwired: 1 out]
        n157 = case shown="True" w347 {
          tunnel: w352 -> [w353 w358]
          tunnel: [w353 w355] -> w351
          frame False {
          }
          frame True {
            n158 = property on="Switch 1 SN" class="CmbBox"(error in=w358) -> (error out=w357:errorcluster, "Value"=w360:string)  [unwired: 1 in, 1 out]
            n159 = property on="SW 1B" class="Knob (strict)"(error in=w357) -> (error out=w356:errorcluster, "Value"=w354:u8)  [unwired: 1 in, 1 out]
            n160 = call "RFSW Set.vi"("RFSW State"=w354, "RFSW Letter"=RFSW_Letter."B", "error in (no error)"=w356, "SN"=w360) -> ("error out"=w355:errorcluster)  [unwired: 4 in, 3 out]
          }
        }
      }
      frame "Set Switch SW2A" {
        # "// Switch 2 is a single pole switch box"
        n161 = property on="Switch 2 SN" class="CmbBox"(error in=w365) -> (error out=w364:errorcluster, "Value"=w366:string)  [unwired: 1 in, 1 out]
        n162 = property on="SW 2A" class="Knob (strict)"(error in=w364) -> (error out=w363:errorcluster, "Value"=w361:u8)  [unwired: 1 in, 1 out]
        n163 = call "RFSW Set.vi"("RFSW State"=w361, "RFSW Letter"=RFSW_Letter."A", "error in (no error)"=w363, "SN"=w366) -> ("error out"=w362:errorcluster)  [unwired: 4 in, 3 out]
      }
      frame "Set Switch SW2B" {
        # "// Switch 2 is a single pole switch box\n// Duplicate this case if station has more than 2 RF switches"
        n164 = local read "Model_Name SW2"() -> (w369:string)
        n165 = Match True/False String(2:"" ("false string"), 3:"RC-2SP6T" ("true string"), 4:w369) -> (0:w368:bool)  [unwired: 1 out]
        n166 = case shown="True" w368 {
          tunnel: w373 -> [w374 w381]
          tunnel: [w374 w380] -> w372
          frame False {
          }
          frame True {
            n167 = property on="Switch 2 SN" class="CmbBox"(error in=w381) -> (error out=w377:errorcluster, "Value"=w378:string)  [unwired: 1 in, 1 out]
            n168 = property on="SW 2A" class="Knob (strict)"(error in=w377) -> (error out=w376:errorcluster, "Value"=w375:u8)  [unwired: 1 in, 1 out]
            n169 = call "RFSW Set.vi"("RFSW State"=w375, "RFSW Letter"=RFSW_Letter."B", "error in (no error)"=w376, "SN"=w378) -> ("error out"=w380:errorcluster)  [unwired: 4 in, 3 out]
          }
        }
      }
      frame "Exit" {
        w384 = TRUE ("force destroy? (F)")
        n170 = Flush Queue(queue=w385, error in (no error)=w382) -> (queue out=w387:refnum<queue>, error out=w386:errorcluster)  [unwired: 1 out]
        n171 = Release Queue(queue=w387, force destroy? (F)=w384, error in (no error)=w386) -> (error out=w383:errorcluster)  [unwired: 2 out]
      }
    }
  }
  n172 = Merge Errors(w15, w5) -> (→"Error Out":errorcluster)
